vi "Translate gRPC Method FullName.vi"(8 "error in (no error)":errorcluster, 11 "Method Full Name in":string) -> (0 "error out":errorcluster, 3 "Method Full Name out":string)   [LabVIEW 2020, in "gRPC Scripting Tools.lvlib"]
uses:
  gRPC Scripting Tools.lvlib
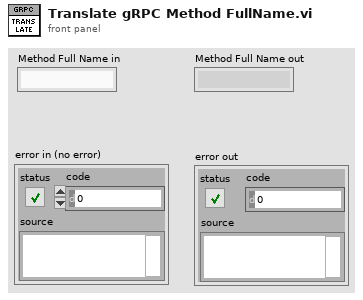
[diagram p1: front panel]
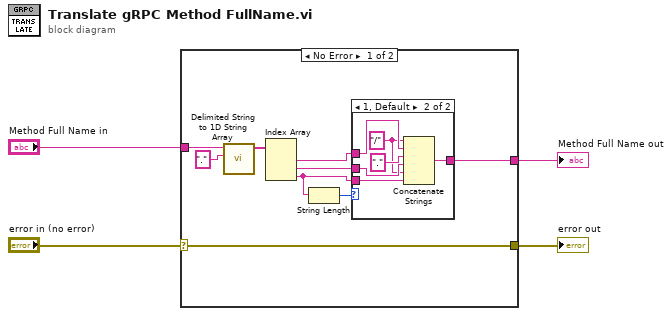
[diagram p0: block diagram]
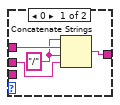
[diagram p2: hidden frame]
diagram:
  n1 = case shown="No Error" "error in (no error)" {
    selector: "error in (no error)" -> [w10 w25]
    tunnel: [w5 w24] -> w4
    tunnel: "Method Full Name in" -> [w12 w24]
    tunnel: [w10 w25] -> w1
    frame No Error {
      n2 = call <vilib>:"Delimited String to 1D String Array.vi"("delimiter"=".", "delimited string"=w12) -> ("string array"=w13:string[])  [unwired: 9 in]
      n3 = Index Array(array=w13) -> (element #1=w7:string, element #2=w6:string, element #3=w9:string)  [unwired: 3 in]
      n4 = String Length(string=w9) -> (length=w8:i32)
      n5 = case shown="1, Default" w8 {
        tunnel: [w17 w23] -> w5
        tunnel: w9 -> [_ w22]
        tunnel: w7 -> [w16 w21]
        tunnel: w6 -> [w14 w20]
        frame 0 {
          w15 = "/" ("string")
          n6 = Concatenate Strings(w15, w16, w15, w14) -> (w17:string)
        }
        frame 1, Default {
          w18 = "/" ("string")
          n7 = Concatenate Strings(w18, w21, "." ("delimiter"), w20, w18, w22) -> (w23:string)
        }
      }
    }
    frame Error {
    }
  }
  "Method Full Name out" <- w4
  "error out" <- w1
